vi "findXMLParentNode.vi"(7 "searchIn":string, 8 "error in (no error)":errorcluster, 9 "type":enum16{"element", "attribute", "value"}(ring), 10 "searchElement":string, 11 "SettingsManager in":refnum<class "SettingsManager.lvclass">) -> (0 "error out":errorcluster, 2 "parentNodePaths":string[](array[string]), 3 "SettingsManager out":refnum<class "SettingsManager.lvclass">)   [LabVIEW 2009, in "Tools.lvlib" / "Settings.lvlib" / "SettingsManager.lvclass"]
uses:
  SettingsManager.lvclass
  SettingsManager.lvclass/SettingsManager.ctl
  xmlNode/xmlNode.lvclass
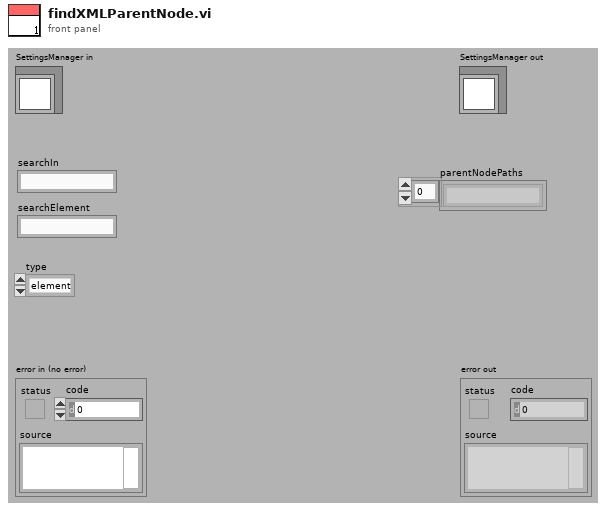
[diagram p1: front panel]
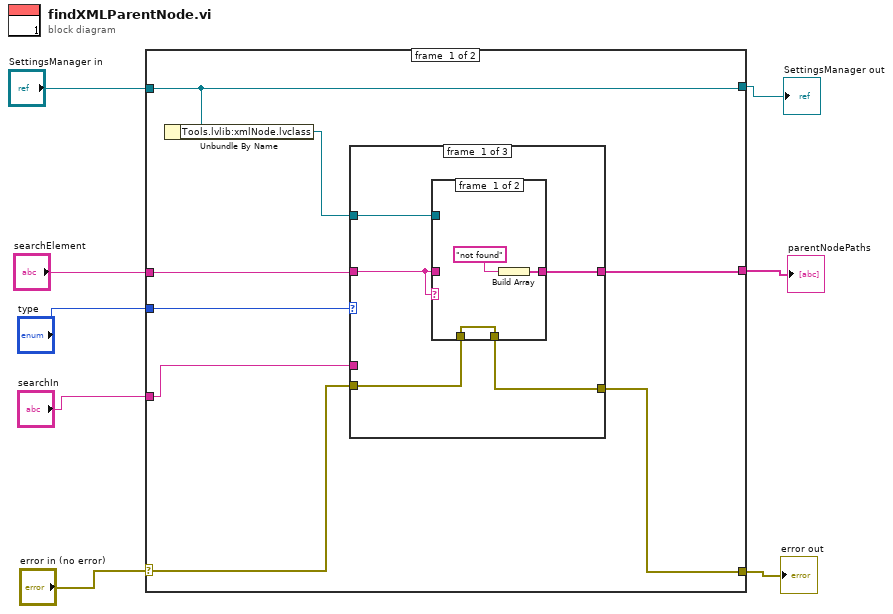
[diagram p0: block diagram]
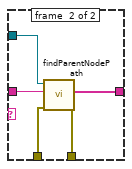
[diagram p2: hidden frame]
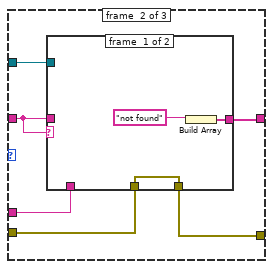
[diagram p3: hidden frame]
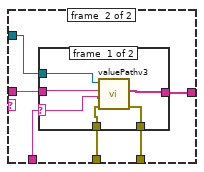
[diagram p4: hidden frame]
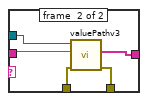
[diagram p5: hidden frame]
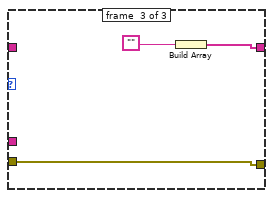
[diagram p6: hidden frame]
diagram:
  n1 = case shown="No Error" "error in (no error)" {
    selector: "error in (no error)" -> [w15 w60]
    tunnel: [w14 w60] -> w7
    tunnel: [w16 w59] -> w5
    tunnel: "SettingsManager in" -> [w16 w59]
    tunnel: "searchElement" -> [w10 _]
    tunnel: "type" -> [w13 _]
    tunnel: [w12 _] -> w2
    tunnel: "searchIn" -> [w9 _]
    frame #0 {
      n2 = Unbundle By Name(w16) -> ("Tools.lvlib:xmlNode.lvclass"=w11:refnum<class "xmlNode.lvclass">)
      n3 = case shown="\"value\"" w13 {
        tunnel: w11 -> [w21 w35 _]
        tunnel: w15 -> [w20 w33 w56]
        tunnel: [w19 w32 w56] -> w14
        tunnel: w10 -> [w17 w31 _]
        tunnel: [w18 w34 w57] -> w12
        tunnel: w9 -> [_ w30 _]
        frame #0 {
          n4 = case shown="Default" w17 {
            tunnel: w21 -> [_ w29]
            tunnel: w20 -> [w22 w28]
            tunnel: [w22 w27] -> w19
            tunnel: w17 -> [_ w26]
            tunnel: [w23 w25] -> w18
            frame #0 {
              n5 = Build Array("not found") -> (w23:string[])
            }
            frame #1 {
              n6 = call-dynamic "findParentNodePath.vi"("error in (no error)"=w28, "searchElement"=w26, "xmlNode in"=w29) -> ("error out"=w27:errorcluster, "Paths"=w25:string[])  [unwired: 6 in, 1 out]
            }
          }
        }
        frame #1 {
          n7 = case shown="Default" w31 {
            tunnel: w35 -> [_ w44]
            tunnel: w31 -> [_ w39]
            tunnel: [w37 w43] -> w34
            tunnel: w33 -> [w36 w42]
            tunnel: [w36 w41] -> w32
            tunnel: w30 -> [_ w40]
            frame #0 {
              n8 = Build Array("not found") -> (w37:string[])
            }
            frame #1 {
              n9 = case shown="Default" w40 {
                selector: w40 -> [w48 _]
                tunnel: w44 -> [w50 w54]
                tunnel: w39 -> [w49 w55]
                tunnel: [w45 w51] -> w43
                tunnel: w42 -> [w47 w53]
                tunnel: [w46 w52] -> w41
                frame #0 {
                  n10 = call-dynamic "valuePathv3.vi"("error in (no error)"=w47, "nodePath"=w48, "value"=w49, "xmlNode in"=w50) -> ("error out"=w46:errorcluster, "Array"=w45:string[])  [unwired: 5 in, 1 out]
                }
                frame #1 {
                  n11 = call-dynamic "valuePathv3.vi"("error in (no error)"=w53, "value"=w55, "xmlNode in"=w54) -> ("error out"=w52:errorcluster, "Array"=w51:string[])  [unwired: 6 in, 1 out]
                }
              }
            }
          }
        }
        frame #2 {
          n12 = Build Array("") -> (w57:string[])
        }
      }
    }
    frame #1 {
    }
  }
  "error out" <- w7
  "SettingsManager out" <- w5
  "parentNodePaths" <- w2
